vi "GenerateFilepath.vi"(8 "error in":errorcluster, 10 "Identifier":string="TestLogger", 11 "Data storage folder":path) -> (0 "error out":errorcluster, 3 "File path out":path)   [LabVIEW 2011, in "Logger.lvclass"]
doc: "Creates the name for the log file for this run with the format (date)_(type of log)((session #)).txt. Puts it in either a wired-in input or in the same folder as the code."
uses:
  Logger.lvclass
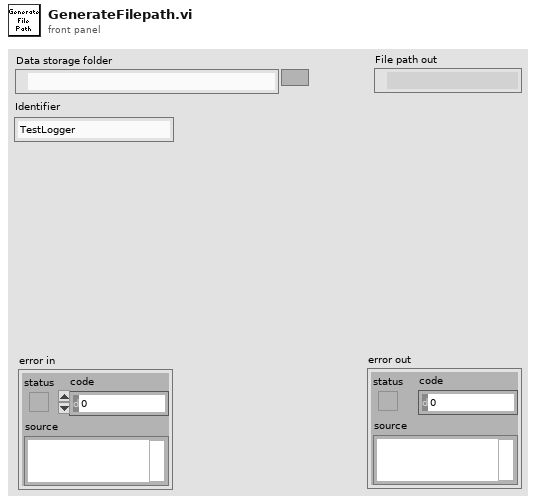
[diagram p1: front panel]
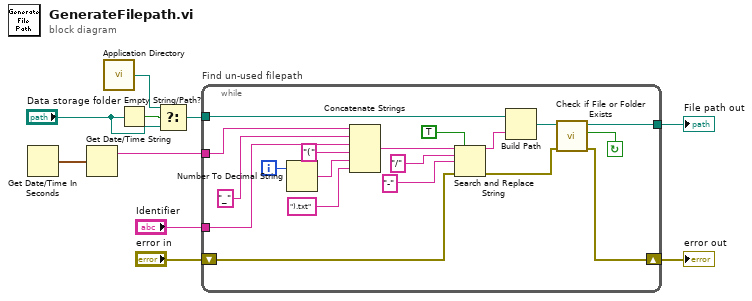
[diagram p0: block diagram]
diagram:
  n1 = Get Date/Time In Seconds() -> (seconds since 1Jan1904=w9:timestamp)
  n2 = Get Date/Time String(seconds (now)=w9) -> (date string=w10:string)  [unwired: 2 in, 1 out]
  n3 = call <vilib>:"Application Directory.vi"() -> ("Application Directory"=w6:path)
  n4 = Empty String/Path?(string/path="Data storage folder") -> (empty?=w1:bool)
  n5 = Select(t=w6, s=w1, f="Data storage folder") -> (s? t:f=w7:path)
  n6 = while "Find un-used filepath" {
    tunnel: w7 -> [w29]
    tunnel: w10 -> [w27]
    shift-right: [w18] -> w5
    shift-left: "error in" -> [w19]
    tunnel: [w16] -> w4
    tunnel: "Identifier" -> [w11]
    i -> [w28]
    stop <- w17 continue-if-true
    n7 = Number To Decimal String(number=w28) -> (decimal integer string=w14:string)  [unwired: 1 in]
    n8 = Concatenate Strings(w27, "_" ("string"), w11, "(" ("string"), w14, ").txt" ("string")) -> (w25:string)
    n9 = Search and Replace String(replace all?=TRUE ("replace all? (F)"), input string=w25, search string="/" ("substring (\"\")"), replace string="-" ("replace string (\"\")"), error in=w19) -> (result string=w20:string, error out=w22:errorcluster)  [unwired: 3 in, 2 out]
    n10 = Build Path(base path=w29, name or relative path=w20) -> (appended path=w26:path)
    n11 = call <vilib>:"Check if File or Folder Exists.vi"("error in (no error)"=w22, "path"=w26) -> ("error out"=w18:errorcluster, "file or folder exists?"=w17:bool, "dup path"=w16:path)  [unwired: 7 in]
  }
  "error out" <- w5
  "File path out" <- w4
